vi "Sort Image File Name.vi"(1 "String1":string, 2 "String2":string) -> (0 "s? t:f":bool)   [LabVIEW 2025]
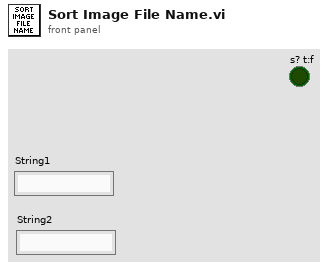
[diagram p1: front panel]
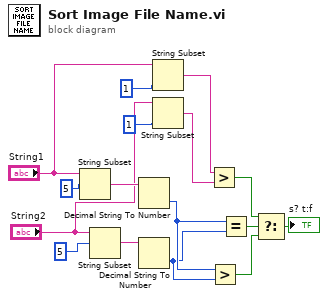
[diagram p0: block diagram]
diagram:
  n1 = String Subset(string="String1", offset (0)=5) -> (substring=w14:string)  [unwired: 1 in]
  n2 = String Subset(string="String2", offset (0)=5) -> (substring=w13:string)  [unwired: 1 in]
  n3 = Decimal String To Number(string=w14) -> (number=w4:i32)  [unwired: 2 in, 1 out]
  n4 = Decimal String To Number(string=w13) -> (number=w3:i32)  [unwired: 2 in, 1 out]
  n5 = String Subset(string="String1", length (rest)=1 ("length (rest)")) -> (substring=w6:string)  [unwired: 1 in]
  n6 = String Subset(string="String2", length (rest)=1 ("length (rest)")) -> (substring=w5:string)  [unwired: 1 in]
  n7 = Greater?(x=w6, y=w5) -> (0:w11:bool)
  n8 = Greater?(x=w4, y=w3) -> (0:w2:bool)
  n9 = Equal?(x=w4, y=w3) -> (x = y?=w12:bool)
  n10 = Select(t=w11, s=w12, f=w2) -> (s? t:f=→"s? t:f":bool)
